vi "Initialize Database.vi"(2 "Error In":errorcluster) -> (0 "Error Out":errorcluster, 1 "Database Connection Out":T1)   [LabVIEW 2020]
uses:
  <vilib>/addons/database/Connection.llb/Conn ObjectReference.ctl
  <vilib>/addons/database/Connection.llb/DB Tools Open Connec (String).vi
  <vilib>/addons/database/NI_Database_API.lvlib
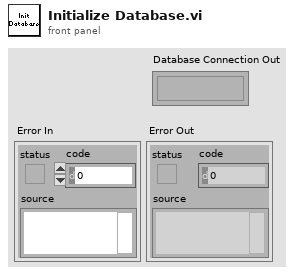
[diagram p1: front panel]
types:
  T1 = typedef "NI_Database_API.lvlib/Conn ObjectReference.ctl" = refnum<k1>
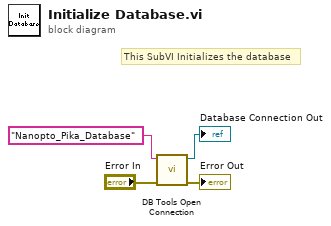
[diagram p0: block diagram]
diagram:
  # "This SubVI Initializes the database"
  n1 = call-poly <vilib>:"DB Tools Open Connection.vi"("error in (no error)"="Error In", "connection information"="Nanopto_Pika_Database") -> ("error out"=→"Error Out":errorcluster, "connection reference"=→"Database Connection Out":T1)  [unwired: 6 in]
